vi "Read Raw Layers.vi"(11 "Image in":refnum<class "Image.lvclass">) -> (2 "Raw Layers":string[](array[string]), 3 "Image out":refnum<class "Image.lvclass">)   [LabVIEW 2017, in "LV Image Editor Framework.lvlib" / "Image.lvclass"]
uses:
  Image.lvclass
  Image.lvclass/Image.ctl
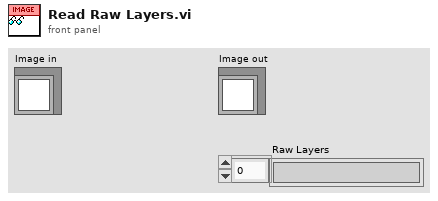
[diagram p1: front panel]
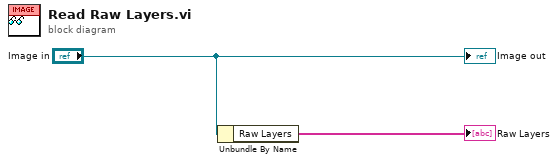
[diagram p0: block diagram]
diagram:
  n1 = Unbundle By Name("Image in") -> ("Raw Layers"=→"Raw Layers":string[])
  "Image out" <- "Image in"
